vi "PH_Beamline.get Vacuum State.vi"(0 "i ref in":refnum<vi>, 2 "Subsystem":T1(ring), 5 "error in (no error)":errorcluster) -> (14 "i ref out":refnum<vi>, 17 "vacua in range":bool, 19 "error out":errorcluster)   [LabVIEW 2014, in "PH_Beamline.lvlib"]
doc: "This VI gets the vacuum state of different subsystems."
uses:
  PH_Beamline.lvlib
  PH_BL-Master/PH_BL-Master.lvlib
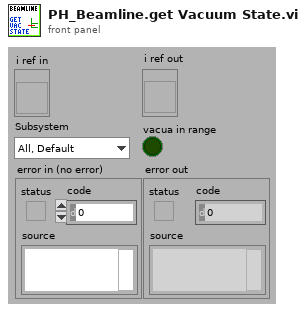
[diagram p1: front panel]
types:
  T1 = enum16{"All, Default", "PreAmp", "MainAmp", "Compressor", "Experiment", "Z6 Telescope"}
  T2 = typedef "PH_BL-Master.lvlib/PH_BL-Master.i attribute.ctl" = cluster{"Remote controlled":bool, "Boolean Condition Service Subscriber":refnum<vi>[], "Picture Condition Service Subscriber":refnum<vi>[], "R2S":cluster{"GUI Ref":refnum<vi>, "State":bool}, "Vacua":cluster{"GUI Ref":refnum<vi>, "Limit":dbl, "Curr Value":dbl, "in range":bool}[], "O2 Inspection":cluster{"GUI Ref":refnum<vi>, "Concentration":dbl, "State":T3}[], "Boolean Status Service Subscriber":cluster{"GUI Ref":refnum<vi>, "Status":T3, "no Link?":bool, "Status Subscriber Class":T4}[], "Picture Status Service Subscriber":cluster{"GUI Ref":refnum<vi>, "Status":T3, "no Link?":bool, "Status Subscriber Class":T4}[], "6P 4Q Service Subscriber":cluster{"GUI Ref":refnum<vi>, "Selector":T5, "no Link?":bool}[], "Index of latest 6P 4Q changing Instance":i32, "Index of latest Picture Status changing Instance":i32, "Index of latest Boolean Status changing Instance":i32, "Vision ID on same Node":string, "Start Phase over?":bool, "GUI Ref Delete":refnum<vi>}
  T3 = typedef "PH_StatusHandler.lvlib/PH_StatusHandler.Status.ctl" = i16
  T4 = typedef "PH_BL-Master.lvlib/PH_BL-Master.Status Subscriber Class.ctl" = enum16{"unknown", "Switch", "BB", "6P Switch", "Switch GUI", "Switch and 6P State", "Force Sensor"}
  T5 = typedef "PH_4_Pos_Selector.lvlib/PH_4_Pos_Selector.Position Selector.ctl" = u16
  T6 = cluster{"GUI Ref":refnum<vi>, "Limit":dbl, "Curr Value":dbl, "in range":bool}[]
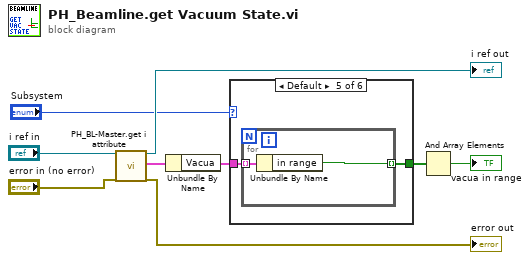
[diagram p0: block diagram]
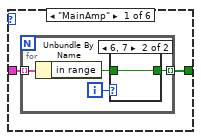
[diagram p2: hidden frame]
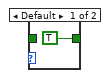
[diagram p3: hidden frame]
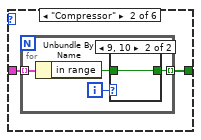
[diagram p4: hidden frame]
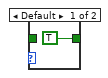
[diagram p5: hidden frame]
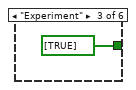
[diagram p6: hidden frame]
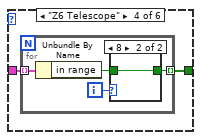
[diagram p7: hidden frame]
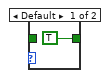
[diagram p8: hidden frame]
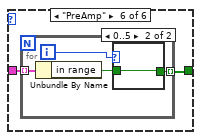
[diagram p9: hidden frame]
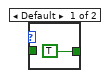
[diagram p10: hidden frame]
diagram:
  n1 = call "PH_BL-Master.get i attribute.vi"("i ref in"="i ref in", "error in (no error)"="error in (no error)") -> ("i ref out"=→"i ref out":refnum<vi>, "i attribute"=w7:T2, "error out"=→"error out":errorcluster)  [unwired: 15 in]
  n2 = Unbundle By Name(w7) -> ("Vacua"=w8:T6)
  n3 = case shown="Default" "Subsystem" {
    tunnel: [w11 w19 bool[] [TRUE] w28 w36 w39] -> w9
    tunnel: w8 -> [w10 w18 _ w27 w35 w40]
    frame "MainAmp" {
      n4 = for {
        tunnel: w10 -> [w15] mode=indexing
        tunnel: [w13] -> w11 mode=indexing
        i -> [w14]
        n5 = Unbundle By Name(w15) -> ("in range"=w12:bool)
        n6 = case shown="6, 7" w14 {
          tunnel: [TRUE ("in range") w17] -> w13
          tunnel: w12 -> [_ w17]
          frame Default {
          }
          frame 6, 7 {
          }
        }
      }
    }
    frame "Compressor" {
      n7 = for {
        tunnel: w18 -> [w23] mode=indexing
        tunnel: [w21] -> w19 mode=indexing
        i -> [w22]
        n8 = Unbundle By Name(w23) -> ("in range"=w20:bool)
        n9 = case shown="9, 10" w22 {
          tunnel: [TRUE ("in range") w25] -> w21
          tunnel: w20 -> [_ w25]
          frame Default {
          }
          frame 9, 10 {
          }
        }
      }
    }
    frame "Experiment" {
    }
    frame "Z6 Telescope" {
      n10 = for {
        tunnel: w27 -> [w32] mode=indexing
        tunnel: [w30] -> w28 mode=indexing
        i -> [w31]
        n11 = Unbundle By Name(w32) -> ("in range"=w29:bool)
        n12 = case shown="8" w31 {
          tunnel: [TRUE ("in range") w34] -> w30
          tunnel: w29 -> [_ w34]
          frame Default {
          }
          frame 8 {
          }
        }
      }
    }
    frame Default {
      n13 = for {
        tunnel: w35 -> [w38] mode=indexing
        tunnel: [w37] -> w36 mode=indexing
        n14 = Unbundle By Name(w38) -> ("in range"=w37:bool)
      }
    }
    frame "PreAmp" {
      n15 = for {
        tunnel: w40 -> [w44] mode=indexing
        tunnel: [w41] -> w39 mode=indexing
        i -> [w43]
        n16 = Unbundle By Name(w44) -> ("in range"=w42:bool)
        n17 = case shown="0..5" w43 {
          tunnel: [TRUE ("in range") w46] -> w41
          tunnel: w42 -> [_ w46]
          frame Default {
          }
          frame 0..5 {
          }
        }
      }
    }
  }
  n18 = And Array Elements(Boolean array=w9) -> (logical AND=→"vacua in range":bool)
